vi "Receive Boolean Value Msg.vi"(8 "error in (no error)":errorcluster, 10 "BooleanValueMsg":refnum<class "BooleanValueMsg.lvclass">, 11 "AutoEventActor in":refnum<class "AutoEventActor.lvclass">) -> (0 "error out":errorcluster, 3 "AutoEventActor out":refnum<class "AutoEventActor.lvclass">)   [LabVIEW 2015, in "ActorAutoRegistration.lvlib" / "AutoEventActor.lvclass"]
uses:
  AutoEventActor.lvclass
  ActorAutoRegistration Messages/BooleanValueMsg/BooleanValueMsg.lvclass
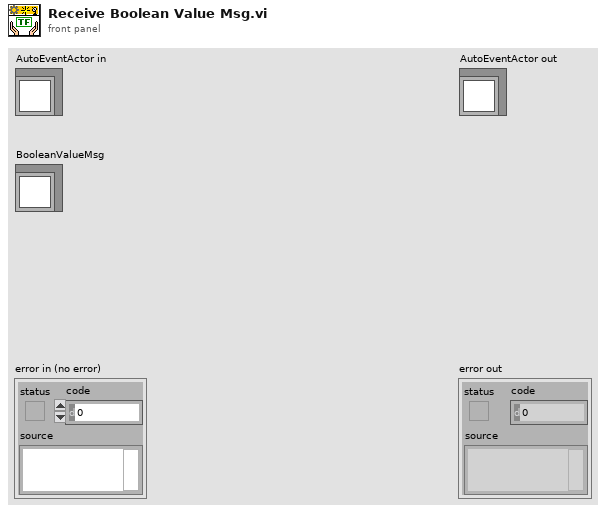
[diagram p1: front panel]
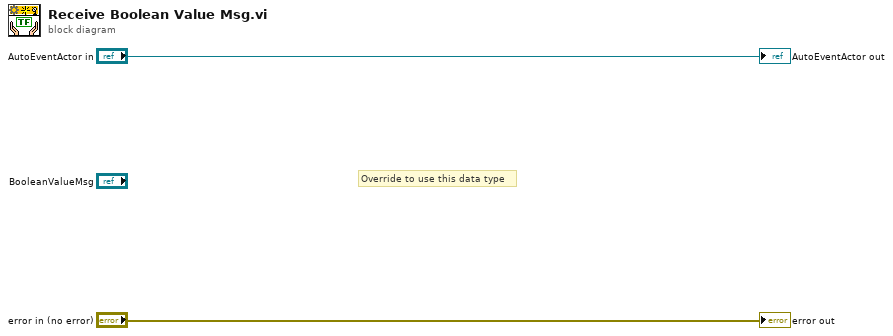
[diagram p0: block diagram]
diagram:
  # "Override to use this data type"
  "error out" <- "error in (no error)"
  "AutoEventActor out" <- "AutoEventActor in"
